vi "Create.vi"(6 "Hooks":T1, 8 "Error In":errorcluster, 11 "Data":refnum<class "Datum.lvclass">) -> (0 "Error Out":errorcluster, 3 "Context":refnum<class "Context.lvclass">)   [LabVIEW 2018, in "Toolkit.lvlib" / "Context.lvclass"]
doc: "Creates a new Context object."
uses:
  Context.lvclass
  Data/Datum/Datum.lvclass
  Hooks/Pre-Render Variable/Render Variable.lvclass
  Context.lvclass/Context.ctl
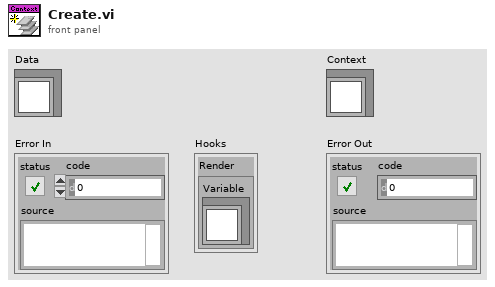
[diagram p1: front panel]
types:
  T1 = cluster{"Render":cluster{"Variable":refnum<class "Render Variable.lvclass">}}
  T2 = cluster{"Variable":refnum<class "Render Variable.lvclass">}
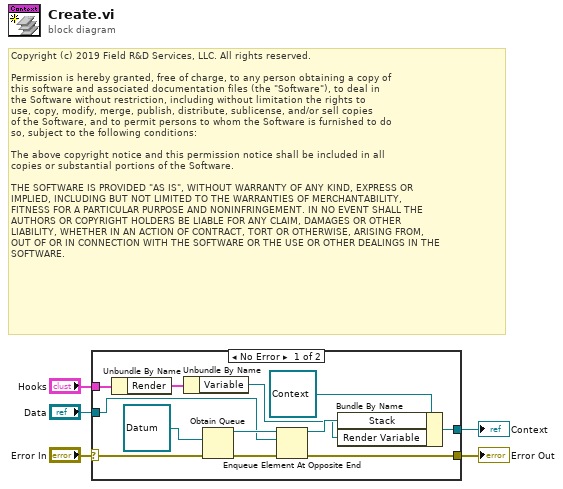
[diagram p0: block diagram]
diagram:
  # "Copyright (c) 2019 Field R&D Services, LLC. All rights reserved.\n\nPermission is hereby granted, free of charge, to any person obtaining a copy of\nthis software and associated documentation files (the \"Software\"), to deal in\nthe Software without restriction, including without limitation the rights to\nuse, copy, modify, merge, publish, distribute, sublicense, and/or sell copies\nof the Software, and to permit persons to whom the Software is furnished to do\nso, subject to the following conditions:\n\nThe above copyright notice and this permission notice shall be included in all\ncopies or substantial portions of the Software.\n\nTHE SOFTWARE IS PROVIDED \"AS IS\", WITHOUT WARRANTY OF ANY KIND, EXPRESS OR\nIMPLIED, INCLUDING BUT NOT LIMITED TO THE WARRANTIES OF MERCHANTABILITY,\nFITNESS FOR A PARTICULAR PURPOSE AND NONINFRINGEMENT. IN NO EVENT SHALL THE\nAUTHORS OR COPYRIGHT HOLDERS BE LIABLE FOR ANY CLAIM, DAMAGES OR OTHER\nLIABILITY, WHETHER IN AN ACTION OF CONTRACT, TORT OR OTHERWISE, ARISING FROM,\nOUT OF OR IN CONNECTION WITH THE SOFTWARE OR THE USE OR OTHER DEALINGS IN THE\nSOFTWARE."
  n1 = case shown="No Error" "Error In" {
    selector: "Error In" -> [w9 w18]
    tunnel: [w14 _] -> w5
    tunnel: [w11 w18] -> w4
    tunnel: "Data" -> [w10 _]
    tunnel: "Hooks" -> [w8 _]
    frame No Error {
      n2 = Unbundle By Name(w8) -> ("Render"=w7:T2)
      n3 = Unbundle By Name(w7) -> ("Variable"=w6:refnum<class "Render Variable.lvclass">)
      n4 = Obtain Queue(element data type=refnum<class "Datum.lvclass"> refnum ("Toolkit.lvlib:Data.lvlib:Abstract.lvclass"), error in (no error)=w9) -> (queue out=w15:refnum<queue>, error out=w12:errorcluster)  [unwired: 3 in, 1 out]
      n5 = Enqueue Element At Opposite End(queue=w15, element=w10, error in (no error)=w12) -> (queue out=w13:refnum<queue>, error out=w11:errorcluster)  [unwired: 1 in, 1 out]
      n6 = Bundle By Name(cluster=refnum<class "Context.lvclass"> refnum ("Toolkit.lvlib:Data.lvlib:Context.lvclass"), "Stack"=w13, "Render Variable"=w6) -> (w14:refnum<class "Context.lvclass">)
    }
    frame Error {
    }
  }
  "Error Out" <- w4
  "Context" <- w5
